vi "CONFIG SPARK MAX PIDF.vi"(0 "MotorControlDevRef":T3, 2 "MOTOR PIDF coefficients":T1={"PIDF"={"P Gain"=0.001, "I Gain"=0.0, "D Gain"=0.0, "F Gain"=0.0012, "I Zone"=0.0, "Min Output"=-1.0, "Max Output"=1.0}, "Smart Motion"={"Max Velocity"=1900.0, "Max Acceleration"=750.0, "Minimum Velocity Output"=0.1, "Allowed Closed Loop Error"=0.02}}, 5 "error in (no error)":errorcluster, 9 "PIDF Slot":i32) -> (14 "MotorControlDevRef OUT":T3, 19 "error out":errorcluster)   [LabVIEW 2023]
uses:
  <vilib>/Rock Robotics/WPI/MotorControl/WPI_MotorControlDeviceRef.ctl
  <vilib>/Rock Robotics/WPI/MotorControl/WPI_MotorControlType.ctl
  <vilib>/Rock Robotics/SystemInterfaces/DIO/FPGA_DIOPWMChannel.ctl
  <vilib>/Rock Robotics/WPI/PWM/WPI_PWMDeadband.ctl
  <vilib>/Rock Robotics/SystemInterfaces/DIO/FPGA_DIOChannel.ctl
  ctrl defs/ctrl motor PIDF coefficients.ctl
  <vilib>/Rock Robotics/WPI/ThirdParty/REV Robotics/REVLib/Typedef/Spark MAX Smart Motion Parameters.ctl
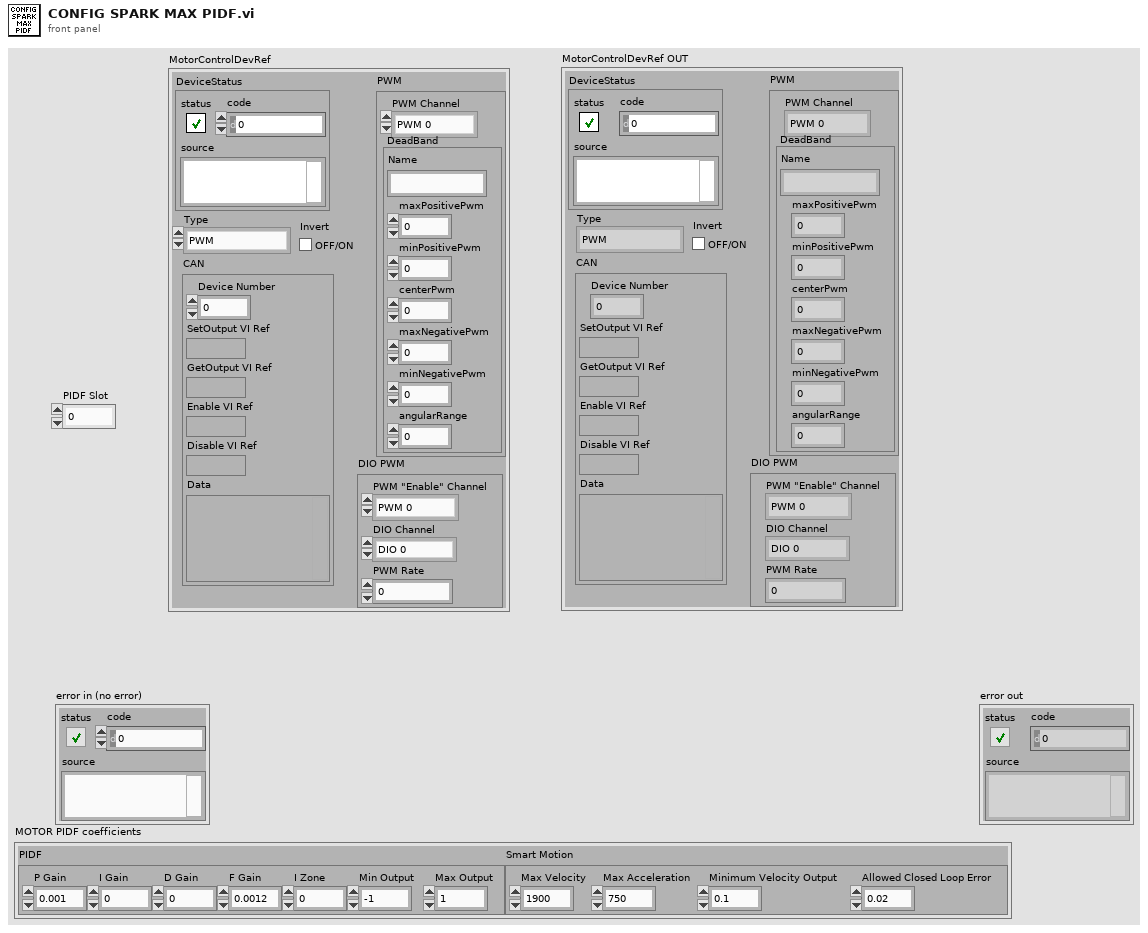
[diagram p1: front panel]
types:
  T1 = typedef "ctrl motor PIDF coefficients.ctl" = cluster{"PIDF":cluster{"P Gain":dbl, "I Gain":dbl, "D Gain":dbl, "F Gain":dbl, "I Zone":dbl, "Min Output":dbl, "Max Output":dbl}, "Smart Motion":T2}
  T2 = typedef "Spark MAX Smart Motion Parameters.ctl" = cluster{"Max Velocity":dbl, "Max Acceleration":dbl, "Minimum Velocity Output":dbl, "Allowed Closed Loop Error":dbl}
  T3 = typedef "WPI_MotorControlDeviceRef.ctl" = cluster{"DeviceStatus":errorcluster, "Type":T4, "PWM":cluster{"PWM Channel":T5, "DeadBand":T6}, "CAN":cluster{"Device Number":u8, "SetOutput VI Ref":variant, "GetOutput VI Ref":variant, "Enable VI Ref":variant, "Disable VI Ref":variant, "Data":variant}, "Invert":bool, "DIO PWM":cluster{"PWM \"Enable\" Channel":T5, "DIOChannel":T7, "PWM Rate":dbl}}
  T4 = typedef "WPI_MotorControlType.ctl" = enum16{"PWM", "CAN", "DIO PWM"}
  T5 = typedef "FPGA_DIOPWMChannel.ctl" = enum8{"PWM 0", "PWM 1", "PWM 2", "PWM 3", "PWM 4", "PWM 5", "PWM 6", "PWM 7", "PWM 8", "PWM 9", "PWM MXP 0", "PWM MXP 1", "PWM MXP 2", "PWM MXP 3", "PWM MXP 4", "PWM MXP 5", "PWM MXP 6", "PWM MXP 7", "PWM MXP 8", "PWM MXP 9", "Invalid"}
  T6 = typedef "WPI_PWMDeadband.ctl" = cluster{"Name":string, "maxPositivePwm":i32, "minPositivePwm":i32, "centerPwm":i32, "maxNegativePwm":i32, "minNegativePwm":i32, "angularRange":u16}
  T7 = typedef "FPGA_DIOChannel.ctl" = enum8{"DIO 0", "DIO 1", "DIO 2", "DIO 3", "DIO 4", "DIO 5", "DIO 6", "DIO 7", "DIO 8", "DIO 9", "DIO MXP 0", "DIO MXP 1", "DIO MXP 2", "DIO MXP 3", "DIO MXP 4", "DIO MXP 5", "DIO MXP 6", "DIO MXP 7", "DIO MXP 8", "DIO MXP 9", "DIO MXP 10", "DIO MXP 11", "DIO MXP 12", "DIO MXP 13", "DIO MXP 14", "DIO MXP 15", "SPI Port CS1", "SPI Port CS2", "SPI Port CS3", "SPI Port MISO", "SPI Port MOSI", "Invalid"}
  T8 = cluster{"P Gain":dbl, "I Gain":dbl, "D Gain":dbl, "F Gain":dbl, "I Zone":dbl, "Min Output":dbl, "Max Output":dbl}
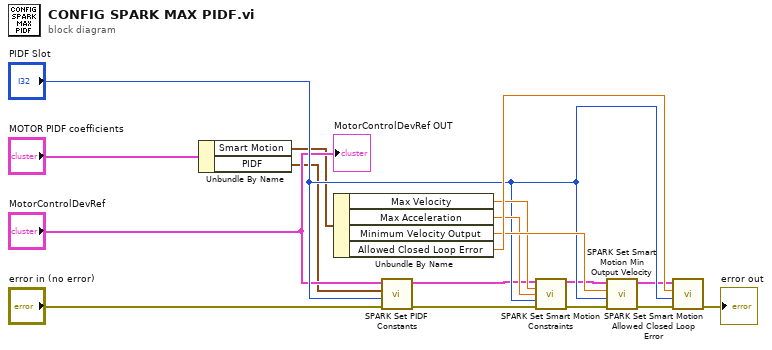
[diagram p0: block diagram]
diagram:
  n1 = Unbundle By Name("MOTOR PIDF coefficients") -> ("Smart Motion"=w2:T2, "PIDF"=w1:T8)
  n2 = Unbundle By Name(w2) -> ("Max Velocity"=w14:dbl, "Max Acceleration"=w15:dbl, "Minimum Velocity Output"=w16:dbl, "Allowed Closed Loop Error"=w17:dbl)
  n3 = call <vilib>:"SPARK Set PIDF Constants.vi"("error in"="error in (no error)", "PIDF Slot"="PIDF Slot", "PID Constants"=w1, "MotorControlDeviceRef"="MotorControlDevRef") -> ("error out"=w7:errorcluster, "MotorControlDeviceRef"=w6:T3)  [unwired: 6 in]
  n4 = call <vilib>:"SPARK Set Smart Motion Constraints.vi"("MotorControlDeviceRef"=w6, "Max Velocity"=w14, "Max Acceleration"=w15, "PIDF Slot (0)"="PIDF Slot", "error in"=w7) -> ("MotorControlDeviceRef"=w9:T3, "error out"=w8:errorcluster)  [unwired: 9 in]
  n5 = call <vilib>:"SPARK Set Smart Motion Min Output Velocity.vi"("error in"=w8, "PIDF Slot (0)"="PIDF Slot", "Minimum Velocity Output"=w16, "MotorControlDeviceRef"=w9) -> ("error out"=w10:errorcluster, "MotorControlDeviceRef"=w11:T3)  [unwired: 6 in]
  n6 = call <vilib>:"SPARK Set Smart Motion Allowed Closed Loop Error.vi"("error in"=w10, "PIDF Slot (0)"="PIDF Slot", "Allowed Closed Loop Error"=w17, "MotorControlDeviceRef"=w11) -> ("error out"=→"error out":errorcluster)  [unwired: 6 in, 1 out]
  "MotorControlDevRef OUT" <- "MotorControlDevRef"
